vi "DtCreateQuadChan.vi"(1 "Clock Prescale":u32=128, 2 "Index Mode":i32(ring)=1400 items=["Disabled"=1400, "Low"=1401, "High"=1402], 3 "X4 Scaling":bool, 5 "Board Name":string, 7 "Quad Decoder Num":u32, 11 "error in (no error)":errorcluster) -> (4 "Task out":i32, 15 "error out":errorcluster)   [LabVIEW 2022 SP3]
doc: "Creates one or more virtual quadrature decoder channels that you can read to determine the current position, in counts, of a quadrature encoder input."
uses:
  DtLvLink.lvlib
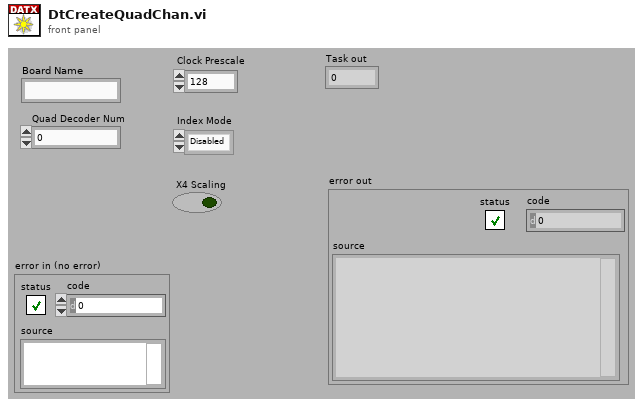
[diagram p1: front panel]
types:
  T1 = enum32{"AnalogInput", "AnalogOutput", "DigitalInput", "DigitalOutput", "Quadrature", "CounterTimer"}
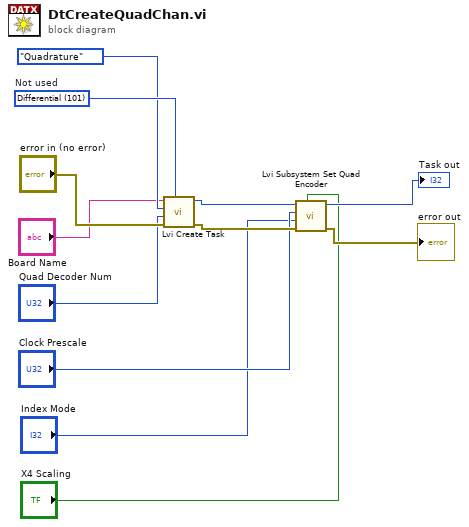
[diagram p0: block diagram]
diagram:
  w12 = 101 items=["SingleEnded"=100, "Differential"=101]  # Not used
  n1 = call "Lvi Create Task.vi"("SEorDiff"=w12, "error in (no error)"="error in (no error)", "SubSysIndex"="Quad Decoder Num", "ChanType"=T1."Quadrature", "BoardName"="Board Name") -> ("error out"=w7:errorcluster, "TaskRef"=w8:i32)  [unwired: 4 in, 1 out]
  n2 = call "Lvi Subsystem Set Quad Encoder.vi"("X4Scaling"="X4 Scaling", "error in (no error)"=w7, "IndexMode"="Index Mode", "ClockPrescale"="Clock Prescale", "TaskRef"=w8) -> ("error out"=→"error out":errorcluster, "TaskRef out"=→"Task out":i32)  [unwired: 4 in, 1 out]
